vi "tm3samp_sequence_electron_wVision.vi"() -> ()   [LabVIEW 2011]
panel:
  out "Photons":sgl format="%.2f"
  out "Display":T1(plugin-control)
  out "Offset":sgl
  out "Coefficient":sgl
  out "Frames Per Second":dbl
  in  "Quit":bool
  out "Error Out":errorcluster
  # "This is an example on how to get\nthe electron count value where \nthe mouse cursor is on the image."
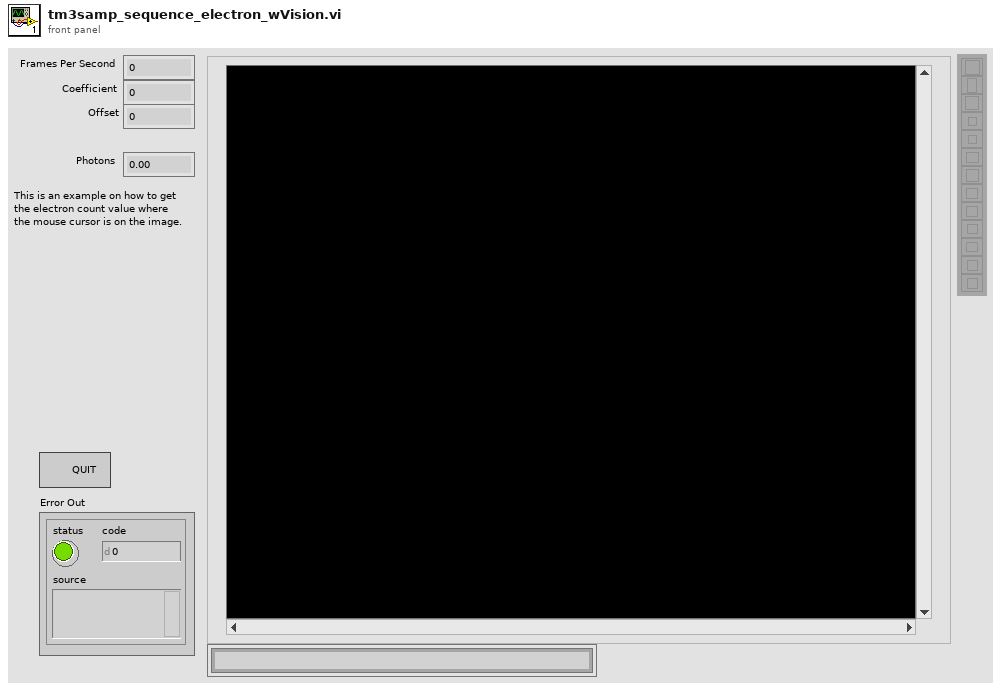
[diagram p1: front panel]
types:
  T1 = typedef "IMAQ Image.ctl" = refnum<image>
  T2 = typedef "Image Type" = u32
  T3 = cluster{"width":u32, "height":u32, "datatype":u32}
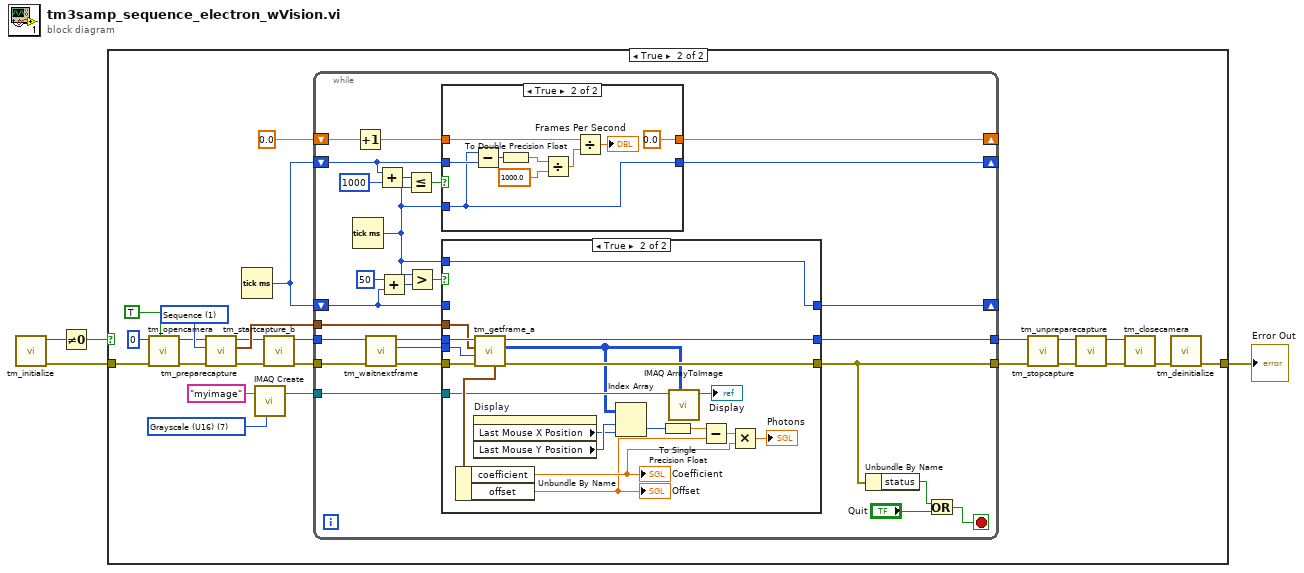
[diagram p0: block diagram]
diagram:
  n1 = call <userlib>:"tm_initialize.vi"() -> ("error out"=w1:errorcluster, "Number Of Cameras"=w2:u32)  [unwired: 10 in]
  n2 = Not Equal To 0?(x=w2) -> (x != 0?=w4:bool)
  n3 = case shown="True" w4 {
    tunnel: w1 -> [w5 w29]
    tunnel: [w5 w26] -> w3
    frame False {
    }
    frame True {
      w9 = T2 7 items=["Grayscale (U8)", "Grayscale (I16)", "Grayscale (SGL)", "Complex (CSG)", "RGB (U32)", "HSL (U32)", "RGB (U64)", "Grayscale (U16)"] ("Image Type")
      w17 = 1 items=["Snap", "Sequence"] ("Capture mode")
      n4 = call <userlib>:"tm_opencamera.vi"("Force Open"=TRUE, "error in (no error)"=w29, "Camera Index"=u32 0) -> ("error out"=w10:errorcluster, "Handle out"=w11:u32)  [unwired: 7 in]
      n5 = call <userlib>:"tm_preparecapture.vi"("error in (no error)"=w10, "Capture mode"=w17, "Handle in"=w11) -> ("error out"=w14:errorcluster, "Buffer"=w16:T3, "Handle out"=w15:u32)  [unwired: 5 in, 1 out]
      n6 = Tick Count (ms)() -> (millisecond timer value=w12:u32)
      n7 = call "IMAQ Create"("Image Name"="myimage", "Image Type"=w9) -> ("New Image"=w8:T1)  [unwired: 3 in, 1 out]
      n8 = call <userlib>:"tm_startcapture_b.vi"("error in (no error)"=w14, "Handle in"=w15) -> ("error out"=w18:errorcluster, "Handle out"=w19:u32)  [unwired: 8 in]
      n9 = while {
        tunnel: [w34] -> w22
        tunnel: [w35] -> w23
        tunnel: w16 -> [w32]
        tunnel: w19 -> [w52]
        tunnel: w18 -> [w53]
        shift-right: [w50] -> _
        shift-left: w12 -> [w47]
        shift-right: [w51] -> _
        shift-left: 0.0 -> [w44]
        shift-right: [w33] -> _
        shift-left: w12 -> [w36]
        tunnel: w8 -> [w31]
        stop <- w30 stop-if-true
        n10 = Tick Count (ms)() -> (millisecond timer value=w37:u32)
        n11 = Increment(x=w44) -> (x+1=w45:dbl)
        n12 = call <userlib>:"tm_waitnextframe.vi"("error in (no error)"=w53, "Handle in"=w52) -> ("error out"=w42:errorcluster, "Frame Index"=w41:i32, "Handle out"=w43:u32)  [unwired: 6 in, 1 out]
        n13 = Add(x=w47, y=u32 1000) -> (x+y=w49:u32)
        n14 = Add(x=u32 50, y=w36) -> (x+y=w39:u32)
        n15 = Less Or Equal?(x=w49, y=w37) -> (x <= y?=w46:bool)
        n16 = Greater?(x=w37, y=w39) -> (0:w38:bool)
        n17 = case shown="True" w46 {
          tunnel: w47 -> [w79 w82]
          tunnel: [w79 w80] -> w50
          tunnel: w45 -> [w78 w86]
          tunnel: w37 -> [_ w80]
          tunnel: [w78 0.0] -> w51
          frame False {
          }
          frame True {
            n18 = Subtract(x=w80, y=w82) -> (x-y=w81:u32)
            n19 = To Double Precision Float(number=w81) -> (double precision float=w88:dbl)
            n20 = Divide(x=w88, y=1000.0) -> (x/y=w85:dbl)
            n21 = Divide(x=w86, y=w85) -> (x/y=→"Frames Per Second":dbl)
          }
        }
        n22 = case shown="True" w38 {
          tunnel: w43 -> [w58 w77]
          tunnel: w42 -> [w57 w76]
          tunnel: w41 -> [_ w75]
          tunnel: w36 -> [w56 _]
          tunnel: w37 -> [_ w74]
          tunnel: [w58 w68] -> w34
          tunnel: [w57 w69] -> w35
          tunnel: [w56 w74] -> w33
          tunnel: w32 -> [_ w73]
          tunnel: w31 -> [_ w71]
          frame False {
          }
          frame True {
            n23 = property on="Display" class="ImageControl"() -> ("Last Mouse X Position"=w59:i32, "Last Mouse Y Position"=w60:i32)  [unwired: 2 in, 2 out]
            n24 = call <userlib>:"tm_getframe_a.vi"("error in (no error)"=w76, "Frame Index"=w75, "Buffer"=w73, "Handle in"=w77) -> ("error out"=w69:errorcluster, "Data 16"=w67:u16[][], "Handle out"=w68:u32, "Electron Info"=w72:cluster{"coefficient":sgl, "offset":sgl})  [unwired: 3 in, 1 out]
            n25 = Unbundle By Name(w72) -> ("coefficient"=w63:sgl, "offset"=w62:sgl)
            "Coefficient" <- w63
            "Offset" <- w62
            n26 = Index Array(array=w67, index (row)=w60, index (col)=w59) -> (element=w65:u16)
            n27 = To Single Precision Float(number=w65) -> (single precision float=w64:sgl)
            n28 = call "IMAQ ArrayToImage"("Image Pixels (U16)"=w67, "Image"=w71) -> ("Image Out"=→"Display":T1)  [unwired: 8 in, 1 out]
            n29 = Subtract(x=w64, y=w62) -> (x-y=w66:sgl)
            n30 = Multiply(x=w66, y=w63) -> (x*y=→"Photons":sgl)
          }
        }
        n31 = Unbundle By Name(w35) -> ("status"=w55:bool)
        n32 = Or(x=w55, y="Quit") -> (x .or. y?=w30:bool)
      }
      n33 = call <userlib>:"tm_stopcapture.vi"("error in (no error)"=w23, "Handle in"=w22) -> ("error out"=w20:errorcluster, "Handle out"=w21:u32)  [unwired: 8 in]
      n34 = call <userlib>:"tm_unpreparecapture.vi"("error in (no error)"=w20, "Handle in"=w21) -> ("error out"=w25:errorcluster, "Handle out"=w24:u32)  [unwired: 8 in]
      n35 = call <userlib>:"tm_closecamera.vi"("error in (no error)"=w25, "Handle in"=w24) -> ("error out"=w27:errorcluster)  [unwired: 9 in]
      n36 = call <userlib>:"tm_deinitialize.vi"("error in (no error)"=w27) -> ("error out"=w26:errorcluster)  [unwired: 10 in]
    }
  }
  "Error Out" <- w3
